vi "FRCts20_WebMethods_Convert_Events_PUT.vi"(8 "error in (no error)":errorcluster, 11 "Single Event in":T3) -> (0 "error out":errorcluster, 3 "Event In":T1)   [LabVIEW 2013, in "FRCts20_WebMethods.lvlib"]
uses:
  FRCts20_WebMethods.lvlib
  Backend/source/VI Source/FRCts20_Backend_API/FRCts20_Backend_API_Event.ctl
  Backend/source/VI Source/FRCts20_Backend_API/FRCts20_Backend_API.lvlib
  Backend/source/VI Source/FRCts20_Backend_API/FRCts20_Backend_API_SW.ctl
  Web Method Public Interface/FRCts20_WebMethods_ctl_teamIdentifier.ctl
  Web Method Public Interface/FRCts20_WebMethods_ctl_singleEvent.ctl
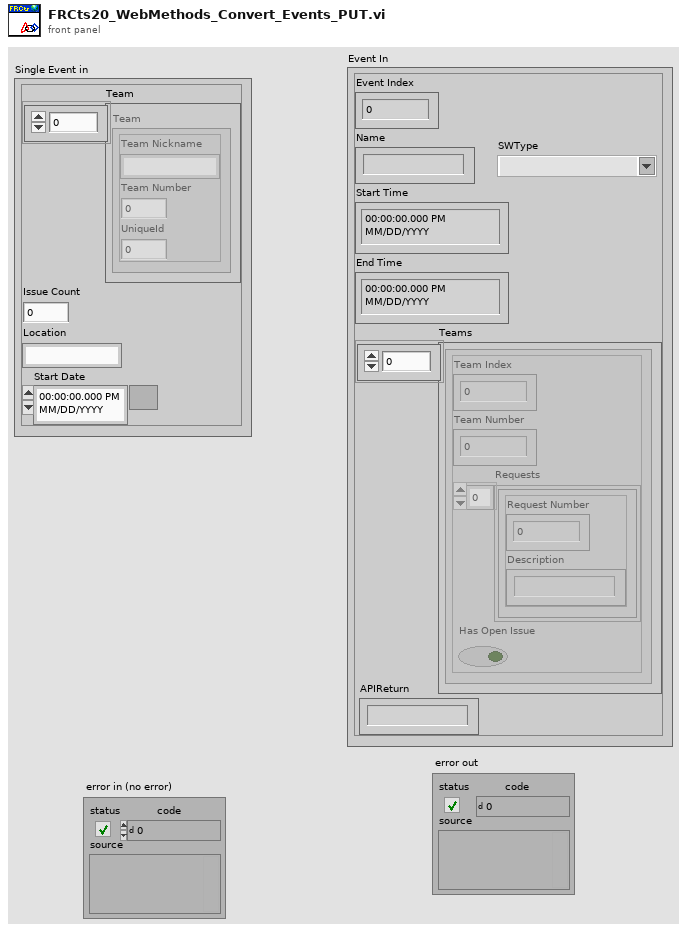
[diagram p1: front panel]
types:
  T1 = typedef "FRCts20_Backend_API.lvlib/FRCts20_Backend_API_Event.ctl" = cluster{"Event Index":u32, "Name":string, "Start Time":timestamp, "End Time":timestamp, "Teams":cluster{"Team Index":u32, "Team Number":u32, "Requests":cluster{"Request Number":u32, "Description":string}[], "Has Open Issue":bool}[], "SWType":T2, "APIReturn":string}
  T2 = typedef "FRCts20_Backend_API.lvlib/FRCts20_Backend_API_SW.ctl" = string
  T3 = typedef "FRCts20_WebMethods.lvlib/FRCts20_WebMethods_ctl_singleEvent.ctl" = cluster{"Team":T4[], "Issue Count":i32, "Location":string, "Start Date ":timestamp}
  T4 = typedef "FRCts20_WebMethods.lvlib/FRCts20_WebMethods_ctl_teamIdentifier.ctl" = cluster{"Team Nickname":string, "Team Number ":u32, "UniqueId":u32}
  T5 = cluster{"Team Index":u32, "Team Number":u32, "Request Number":u32, "Description":string, "Has Open Issue":bool}
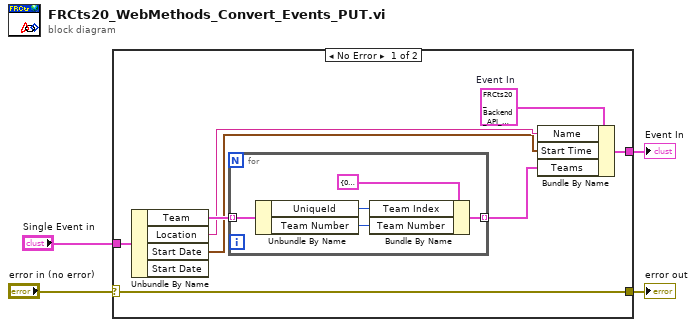
[diagram p0: block diagram]
diagram:
  n1 = case shown="No Error" "error in (no error)" {
    selector: "error in (no error)" -> [w9 w18]
    tunnel: [w9 w18] -> w3
    tunnel: "Single Event in" -> [w12 _]
    tunnel: [w10 _] -> w1
    frame No Error {
      w11 = T1 {"Event Index"=0, "Name"="", "Start Time"=timestamp(0 s since 1904-01-01), "End Time"=timestamp(0 s since 1904-01-01), "Teams"=[], "SWType"="", "APIReturn"=""}  # Event In
      n2 = Unbundle By Name(w12) -> ("Team"=w8:T4[], "Location"=w6:string, "Start Date"=w5:timestamp)  [unwired: 1 out]
      n3 = for {
        tunnel: w8 -> [w17] mode=indexing
        tunnel: [w13] -> w7 mode=indexing
        n4 = Unbundle By Name(w17) -> ("UniqueId"=w15:u32, "Team Number"=w14:u32)
        n5 = Bundle By Name(cluster=T5 {"Team Index"=0, "Team Number"=0, "Request Number"=0, "Description"="", "Has Open Issue"=FALSE} ("Team"), "Team Index"=w15, "Team Number"=w14) -> (w13:T5)
      }
      n6 = Bundle By Name(cluster=w11, "Name"=w6, "Start Time"=w5, "Teams"=w7) -> (w10:T1)
    }
    frame Error {
    }
  }
  "Event In" <- w1
  "error out" <- w3
